vi "I2C LJTick-DAC DACA.vi"() -> ()   [LabVIEW 2020]
panel:
  out "Read Names":string[](array[string])
  out "Read Values":dbl[](array[numeric])
  out "Error String":string
  out "ConnectionType Out":i32
  out "DeviceType Out":i32
  in  "Identifier":string="LJM_idANY"
  in  "ConnectionType":string="LJM_ctANY"
  in  "DeviceType":string="LJM_dtANY"
  out "error out":errorcluster
  # "Before running this program:\n1. Attach a LJTick-DAC to FIO0 and FIO1\n2. Attach a wire between the screw terminal \nlabeled DACA on the LJTick-DAC and AIN0\n\nProgram sets the DACA output on the LJTick-DAC \nwith a raw value (0-65535), roughly -10V to 10V \nand reads the voltage on AIN0.\n\nAlso note, the value reported for I2C_ACKS will be \ngreater than zero if the LJTick-DAC is connected \nproperly."
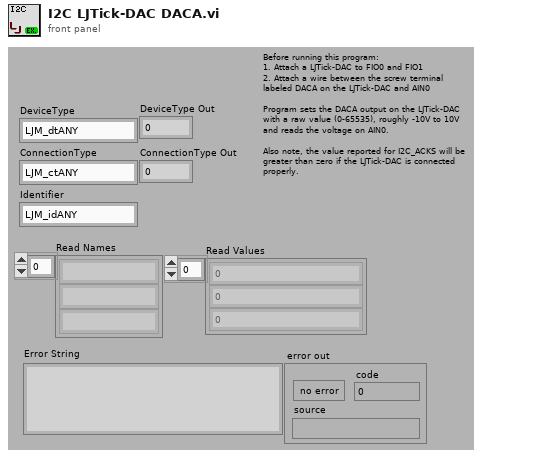
[diagram p1: front panel]
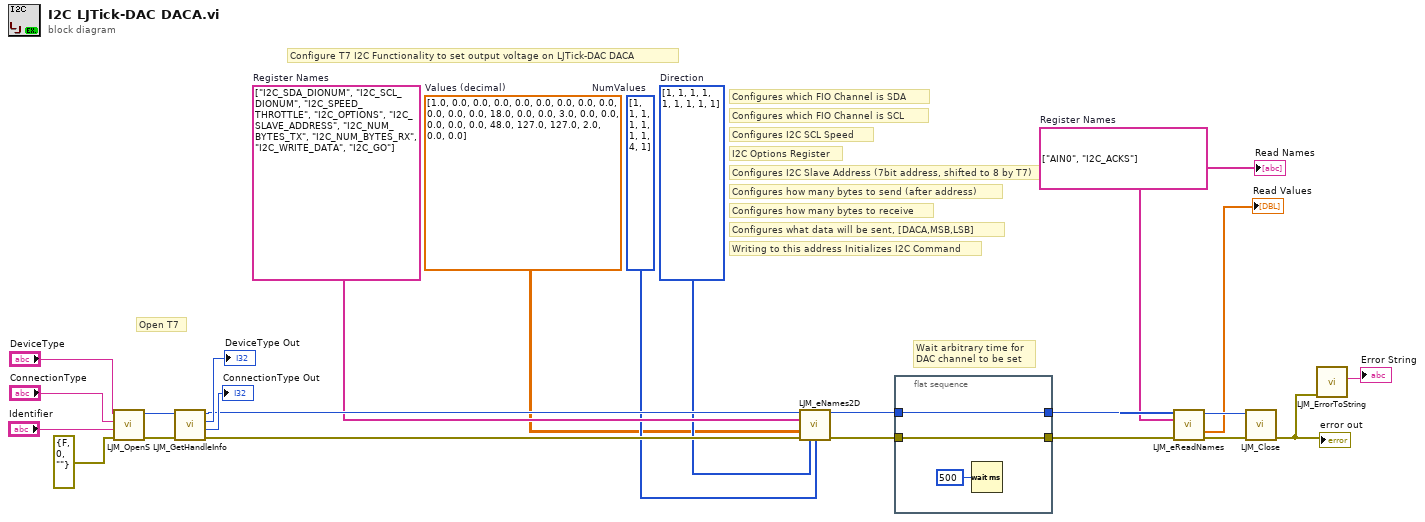
[diagram p0: block diagram]
diagram:
  w1 = dbl[][] [[1.0, 0.0, 0.0], [0.0, 0.0, 0.0], [0.0, 0.0, 0.0], [0.0, 0.0, 0.0], [18.0, 0.0, 0.0], [3.0, 0.0, 0.0], [0.0, 0.0, 0.0], [48.0, 127.0, 127.0], [2.0, 0.0, 0.0]]  # Values (decimal)
  w2 = i32[] [1, 1, 1, 1, 1, 1, 1, 1, 1] items=["Read", "Write"]  # Direction
  w3 = i32[] [1, 1, 1, 1, 1, 1, 1, 4, 1]  # NumValues
  w12 = string[] ["AIN0", "I2C_ACKS"]  # Register Names
  w4 = string[] ["I2C_SDA_DIONUM", "I2C_SCL_DIONUM", "I2C_SPEED_THROTTLE", "I2C_OPTIONS", "I2C_SLAVE_ADDRESS", "I2C_NUM_BYTES_TX", "I2C_NUM_BYTES_RX", "I2C_WRITE_DATA", "I2C_GO"]  # Register Names
  # "Wait arbitrary time for \nDAC channel to be set"
  # "Configures which FIO Channel is SDA"
  # "Configures which FIO Channel is SCL"
  # "Configures I2C SCL Speed"
  # "I2C Options Register"
  # "Configures I2C Slave Address (7bit address, shifted to 8 by T7)"
  # "Configures how many bytes to send (after address)"
  # "Configures how many bytes to receive"
  # "Configures what data will be sent, [DACA,MSB,LSB]"
  # "Writing to this address Initializes I2C Command"
  # "Open T7"
  # "Configure T7 I2C Functionality to set output voltage on LJTick-DAC DACA"
  n1 = call "LJM_OpenS.vi"("error in"=errorcluster {"status"=FALSE, "code"=0, "source"=""} ("error in (no error)"), "Identifier"="Identifier", "ConnectionType"="ConnectionType", "DeviceType"="DeviceType") -> ("error out"=w23:errorcluster, "Handle"=w22:i32)  [unwired: 6 in]
  n2 = call "LJM_GetHandleInfo.vi"("error in"=w23, "Handle In"=w22) -> ("error out"=w8:errorcluster, "ConnectionType"=→"ConnectionType Out":i32, "DeviceType"=→"DeviceType Out":i32, "Handle Out"=w5:i32)  [unwired: 2 in, 4 out]
  n3 = call "LJM_eNames2D.vi"("Handle In"=w5, "aNames"=w4, "aValuesIn"=w1, "error in"=w8, "aWrites"=w2, "aNumValues"=w3) -> ("Handle Out"=w6:i32, "error out"=w7:errorcluster)  [unwired: 6 in, 2 out]
  n4 = flat-sequence {
    tunnel: w7 -> [w26]
    tunnel: w6 -> [w27]
    tunnel: [w27] -> w10
    tunnel: [w26] -> w9
    frame #0 {
      n5 = Wait (ms)(milliseconds to wait=u32 500) -> ()  [unwired: 1 out]
    }
  }
  n6 = call "LJM_eReadNames.vi"("Handle In"=w10, "aNames"=w12, "error in"=w9) -> ("Handle Out"=w13:i32, "aValuesOut"=→"Read Values":dbl[], "error out"=w14:errorcluster)  [unwired: 9 in, 1 out]
  n7 = call "LJM_Close.vi"("error in"=w14, "Handle"=w13) -> ("error out"=w16:errorcluster)  [unwired: 9 in]
  "error out" <- w16
  n8 = call "LJM_ErrorToString.vi"("error in"=w16) -> ("String"=→"Error String":string)  [unwired: 10 in]
  "Read Names" <- w12
